vi "Actor Core.vi"(8 "error in":errorcluster, 11 "Main Window in":refnum<class "Main Window.lvclass">) -> (0 "error out":errorcluster, 3 "Actor out":refnum<class "Actor.lvclass">)   [LabVIEW 2021, in "Recipe.lvlib" / "Main Window.lvclass"]
doc: "The user interface for this panel.\n\n----\nPlease see the following web address for additional documentation and tutorial information:\nhttp://www.mooregoodideas.com/mgi-panel-manager/\n\nAuthor: Derek Trepanier\n\nCopyright (c) 2018, Moore Good Ideas, Inc.\n\nAll rights reserved.\n\nRedistribution and use in source and binary forms, with or without modification, are permitted provided that the following conditions are met:\n\n * Redistributions of source code must retain the above copyright notice, this list of conditions and the following disclaimer.\n * Redistributions in binary form must reproduce the above copyright notice, this list of conditions and the following disclaimer in the documentation and/or other materials provided with the distribution.\n * Neither the name of Moore Good Ideas, Inc. nor the names of its contributors may be used to endorse or promote products derived from this software without specific prior written permission.\n\nTHIS SOFTWARE IS PROVIDED BY THE COPYRIGHT HOLDERS AND CONTRIBUTORS \"AS IS\" AND ANY EXPRESS OR IMPLIED WARRANTIES, INCLUDING, BUT NOT LIMITED TO, THE IMPLIED WARRANTIES OF MERCHANTABILITY AND FITNESS FOR A PARTICULAR PURPOSE ARE DISCLAIMED. IN NO EVENT SHALL THE COPYRIGHT OWNER OR CONTRIBUTORS BE LIABLE FOR ANY DIRECT, INDIRECT, INCIDENTAL, SPECIAL, EXEMPLARY, OR CONSEQUENTIAL DAMAGES (INCLUDING, BUT NOT LIMITED TO, PROCUREMENT OF SUBSTITUTE GOODS OR SERVICES; LOSS OF USE, DATA, OR PROFITS; OR BUSINESS INTERRUPTION) HOWEVER CAUSED AND ON ANY THEORY OF LIABILITY, WHETHER IN CONTRACT, STRICT LIABILITY, OR TORT (INCLUDING NEGLIGENCE OR OTHERWISE) ARISING IN ANY WAY OUT OF THE USE OF THIS SOFTWARE, EVEN IF ADVISED OF THE POSSIBILITY OF SUCH DAMAGE."
uses:
  Main Window.lvclass
  C:/Program Files (x86)/National Instruments/LabVIEW 2021/vi.lib/MGI/Panel Manager/Panel Actor/Panel Actor/Panel Actor.lvclass
  <vilib>/ActorFramework/Actor/Actor.lvclass
  Main Window.lvclass/Main Window.ctl
  <vilib>/ActorFramework/Message Enqueuer/Message Enqueuer.lvclass/Message Enqueuer.ctl
  Main Window Messages/Show Recipe Msg/Show Recipe Msg.lvclass/Show Recipe Msg.ctl
  <vilib>/ActorFramework/Message Enqueuer/Enqueue.vi
  <vilib>/ActorFramework/Stop Msg/Stop Msg.lvclass
  C:/Program Files (x86)/National Instruments/LabVIEW 2021/vi.lib/ActorFramework/Message/Message.lvclass
  Main Window Messages/New Recipe Window Msg/New Recipe Window Msg.lvclass
  Main Window Messages/Show Recipe Msg/Show Recipe Msg.lvclass
  <vilib>/ActorFramework/Message Priority Queue/Priority Enqueue.vi
  <vilib>/MGI/Panel Manager/Panel Actor/Panel Actor/Panel Actor.lvclass
  Windows/System32/user32.dll
panel:
  in  "New Recipe":bool
  in  "Header Button":bool
  in  "Header Button 2":bool
  in  "Window Maximize":bool
  in  "Window Minimize":bool
  in  "Close":bool
  in  "Recipe List":i32(listbox)
  # "Recipe"
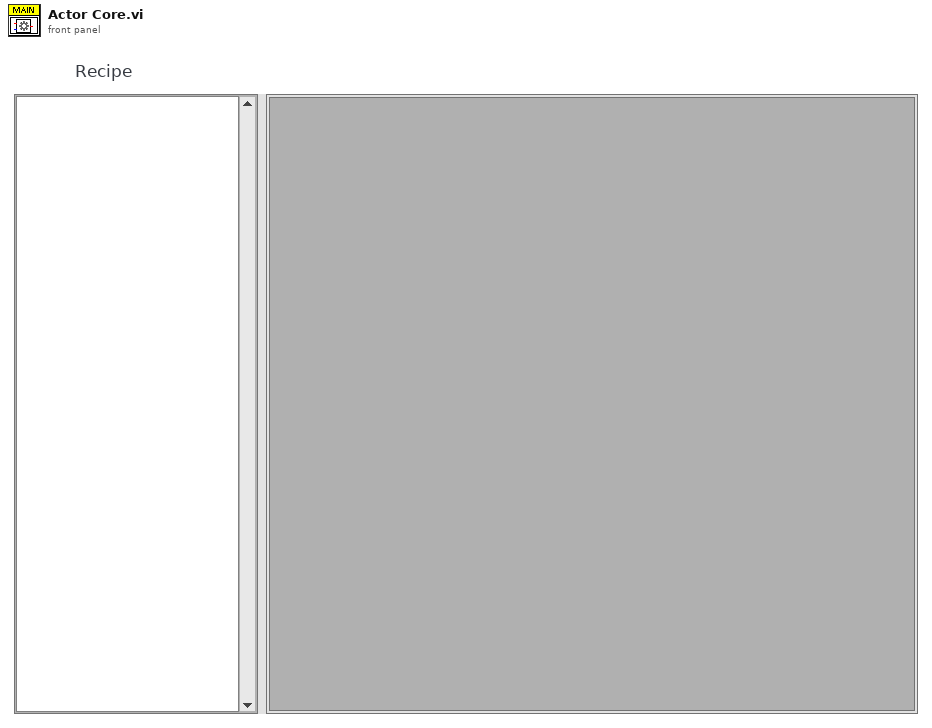
[diagram p1: front panel]
types:
  T1 = enum32{"Invalid", "Standard", "Closed", "Hidden", "Minimized", "Maximized"}
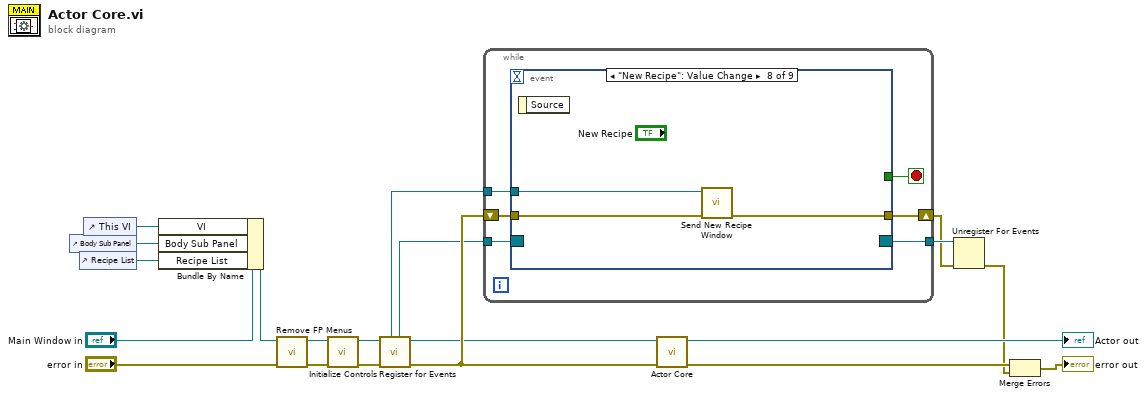
[diagram p0: block diagram]
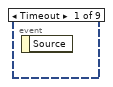
[diagram p2: hidden frame]
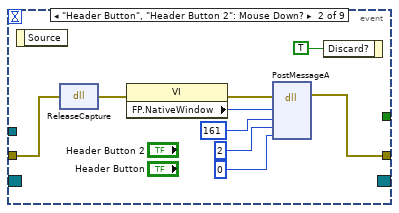
[diagram p3: hidden frame]
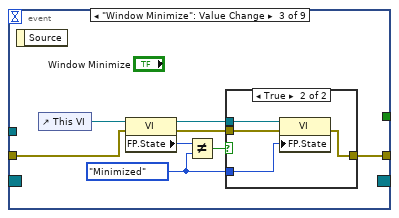
[diagram p4: hidden frame]
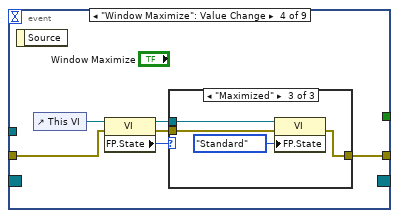
[diagram p6: hidden frame]
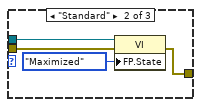
[diagram p8: hidden frame]
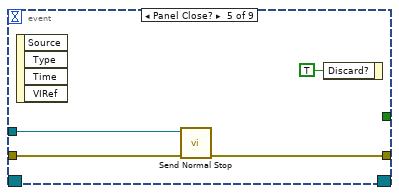
[diagram p9: hidden frame]
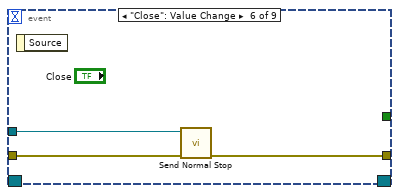
[diagram p10: hidden frame]
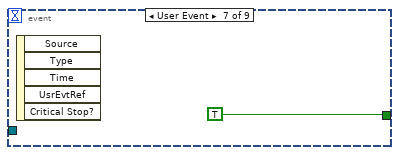
[diagram p11: hidden frame]
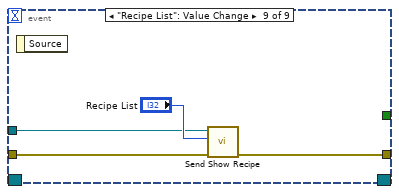
[diagram p12: hidden frame]
diagram:
  n1 = control-ref of="Body Sub Panel"() -> (w10:refnum<vi>)
  n2 = control-ref of="Recipe List"() -> (w6:refnum<vi>)
  n3 = control-ref of="This VI"() -> (w9:refnum<vi>)
  n4 = Bundle By Name(cluster="Main Window in", "VI"=w9, "Body Sub Panel"=w10, "Recipe List"=w6) -> (w7:refnum<class "Main Window.lvclass">)
  n5 = call "Remove FP Menus.vi"("error in (no error)"="error in", "Main Window in"=w7) -> ("error out"=w8:errorcluster, "Main Window out"=w4:refnum<class "Main Window.lvclass">)  [unwired: 8 in]
  n6 = call "Initialize Controls.vi"("error in (no error)"=w8, "Main Window in"=w4) -> ("error out"=w5:errorcluster, "Main Window out"=w3:refnum<class "Main Window.lvclass">)  [unwired: 8 in]
  n7 = call <vilib>:"Register for Events.vi"("Error In"=w5, "Panel Actor in"=w3) -> ("Error Out"=w20:errorcluster, "Panel Actor out"=w17:refnum<class "Main Window.lvclass">, "Pnl Actor"=w16:refnum<event-registration>, "Self Enqueuer"=w15:refnum<class "Message Enqueuer.lvclass">)  [unwired: 6 in]
  n8 = while {
    tunnel: w16 -> [w26]
    tunnel: w15 -> [w25]
    shift-right: [w23] -> w12
    shift-left: w20 -> [w22]
    tunnel: [w21] -> w14
    stop <- w24 stop-if-true
    n9 = event shown="[7] \"New Recipe\": Value Change" {
      selector: w26 -> [_ _ _ _ _ _ _ _ _]
      dyn-events: [_ _ _ _ _ _ _ _ _] -> w21
      timeout: _ -> [_ _ _ _ _ _ _ _ _]
      tunnel: w25 -> [_ _ _ _ w66 w70 _ w74 w77]
      tunnel: [_ _ _ _ _ _ TRUE _ _] -> w24
      tunnel: [_ w30 w36 w50 w65 w68 _ w72 w75] -> w23
      tunnel: w22 -> [_ w34 w37 w53 w64 w69 _ w73 w76]
      event Timeout {
        n10 = event-data() -> ()  [unwired: 1 in, 1 out]
      }
      event "Header Button", "Header Button 2": Mouse Down? {
        n11 = event-data() -> ()  [unwired: 1 in, 1 out]
        n12 = dll-call lib="C:/Windows/System32/user32.dll" fn="ReleaseCapture"(error in=w34) -> (error out=w33:errorcluster)  [unwired: 3 in, 1 out]
        n13 = property class="VI"(error in=w33) -> (error out=w32:errorcluster, "FP.NativeWindow"=w31:u64)  [unwired: 1 in, 1 out]
        n14 = dll-call lib="C:/Windows/System32/user32.dll" fn="PostMessageA"(error in=w32, "arg1"=w31, "arg2"=161, "arg3"=2, "arg4"=0) -> (error out=w30:errorcluster)  [unwired: 7 in, 1 out]
        n15 = event-data("Discard?"=TRUE) -> ()  [unwired: 1 in, 1 out]
      }
      event "Window Minimize": Value Change {
        w39 = T1."Minimized" ("Front Panel Window:State")
        n16 = event-data() -> ()  [unwired: 1 in, 1 out]
        n17 = control-ref of="This VI"() -> (w42:refnum<vi>)
        n18 = property class="VI"(reference=w42, error in=w37) -> (reference out=w43:refnum<vi>, error out=w38:errorcluster, "FP.State"=w41:T1)
        n19 = Not Equal?(x=w41, y=w39) -> (x != y?=w40:bool)
        n20 = case shown="True" w40 {
          tunnel: w43 -> [_ w48]
          tunnel: w39 -> [_ w47]
          tunnel: w38 -> [w44 w46]
          tunnel: [w44 w45] -> w36
          frame False {
          }
          frame True {
            n21 = property class="VI"(reference=w48, error in=w46, "FP.State"=w47) -> (error out=w45:errorcluster)  [unwired: 1 out]
          }
        }
      }
      event "Window Maximize": Value Change {
        n22 = event-data() -> ()  [unwired: 1 in, 1 out]
        n23 = control-ref of="This VI"() -> (w52:refnum<vi>)
        n24 = property class="VI"(reference=w52, error in=w53) -> (reference out=w54:refnum<vi>, error out=w51:errorcluster, "FP.State"=w49:T1)
        n25 = case shown="\"Maximized\"" w49 {
          tunnel: w54 -> [_ w59 w63]
          tunnel: w51 -> [w55 w58 w62]
          tunnel: [w55 w57 w61] -> w50
          frame Default {
          }
          frame "Standard" {
            n26 = property class="VI"(reference=w59, error in=w58, "FP.State"=T1."Maximized" ("Front Panel Window:State")) -> (error out=w57:errorcluster)  [unwired: 1 out]
          }
          frame "Maximized" {
            n27 = property class="VI"(reference=w63, error in=w62, "FP.State"=T1."Standard" ("Front Panel Window:State")) -> (error out=w61:errorcluster)  [unwired: 1 out]
          }
        }
      }
      event Panel Close? {
        n28 = event-data() -> ()  [unwired: 1 in, 4 out]
        n29 = call <vilib>:"Send Normal Stop.vi"("error in (no error)"=w64, "Message Enqueuer"=w66) -> ("error out"=w65:errorcluster)  [unwired: 9 in]
        n30 = event-data("Discard?"=TRUE) -> ()  [unwired: 1 in, 1 out]
      }
      event "Close": Value Change {
        n31 = event-data() -> ()  [unwired: 1 in, 1 out]
        n32 = call <vilib>:"Send Normal Stop.vi"("error in (no error)"=w69, "Message Enqueuer"=w70) -> ("error out"=w68:errorcluster)  [unwired: 9 in]
      }
      event User Event {
        n33 = event-data() -> ()  [unwired: 1 in, 5 out]
      }
      event "New Recipe": Value Change {
        n34 = event-data() -> ()  [unwired: 1 in, 1 out]
        n35 = call "Send New Recipe Window.vi"("error in (no error)"=w73, "Message Enqueuer"=w74) -> ("error out"=w72:errorcluster)  [unwired: 8 in, 1 out]
      }
      event "Recipe List": Value Change {
        n36 = event-data() -> ()  [unwired: 1 in, 1 out]
        n37 = call "Send Show Recipe.vi"("error in (no error)"=w76, "List Index"="Recipe List", "Message Enqueuer"=w77) -> ("error out"=w75:errorcluster)  [unwired: 7 in, 1 out]
      }
    }
  }
  n38 = call-parent "Actor Core.vi"("error in"=w20, "Panel Actor in"=w17) -> ("error out"=w19:errorcluster, "Actor out"=→"Actor out":refnum<class "Actor.lvclass">)  [unwired: 8 in]
  n39 = Unregister For Events(event registration refnum=w14, error in=w12) -> (error out=w11:errorcluster)
  n40 = Merge Errors(w19, w11) -> (→"error out":errorcluster)
